vi "Property Node (niFile).vi"   [LabVIEW 2020, in "niSkylineFileIngestion.lvlib"]
doc: "Provides information about an open file reference."
uses:
  niSkylineFileIngestion.lvlib
  Base/NI Skyline File Base.lvclass
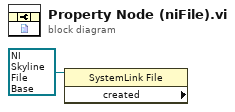
[diagram p0: block diagram]
diagram:
  n1 = property class="SystemLink File" props=["created"](reference=refnum<class "NI Skyline File Base.lvclass"> refnum) -> ()  [unwired: 1 in, 3 out]
